vi "update anott. name.vi"(8 "error in (no error)":errorcluster, 9 "Annotation No":i32, 10 "Name":string, 11 "XYGraph in":refnum<vi>) -> (0 "error out":errorcluster, 3 "XYGraph out":refnum<vi>)   [LabVIEW 2014]
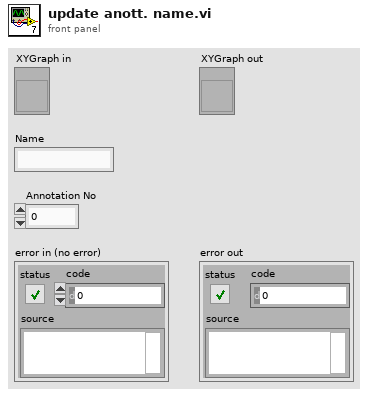
[diagram p1: front panel]
types:
  T1 = typedef "LVAnnotationListTypeDef.ctl" = cluster{"Name":string, "Color":u32, "Style":u8, "Point Style":u8, "Name Visible":bool, "Allow Drag":bool, "Annotation Mode":u32, "Plot":i32, "Index":i32, "Position":cluster{"X":dbl, "Y":dbl}, "X Scale":u32, "Y Scale":u32, "Show Arrow":bool, "Lock Name":bool, "Plot Area":i32, "Label Offset":cluster{"X":dbl, "Y":dbl}}[]
  T2 = cluster{"Name":string, "Color":u32, "Style":u8, "Point Style":u8, "Name Visible":bool, "Allow Drag":bool, "Annotation Mode":u32, "Plot":i32, "Index":i32, "Position":cluster{"X":dbl, "Y":dbl}, "X Scale":u32, "Y Scale":u32, "Show Arrow":bool, "Lock Name":bool, "Plot Area":i32, "Label Offset":cluster{"X":dbl, "Y":dbl}}
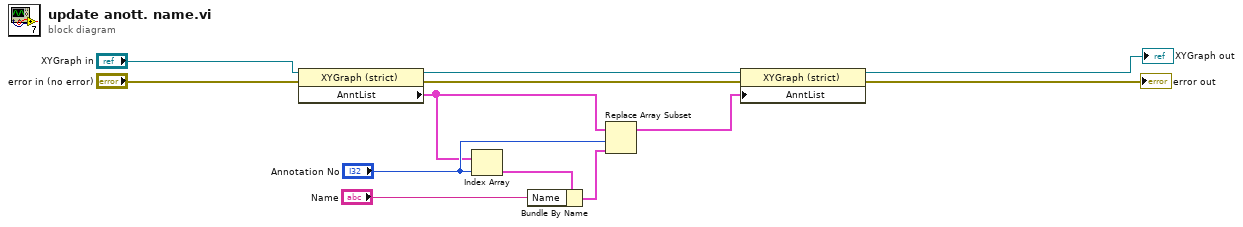
[diagram p0: block diagram]
diagram:
  n1 = property class="XYGraph (strict)"(reference="XYGraph in", error in="error in (no error)") -> (reference out=w8:refnum<vi>, error out=w7:errorcluster, "AnntList"=w4:T1)
  n2 = Index Array(array=w4, index="Annotation No") -> (element=w9:T2)
  n3 = Bundle By Name(cluster=w9, "Name"="Name") -> (w10:T2)
  n4 = Replace Array Subset "Replace Array Subset"(array=w4, new element=w10, index="Annotation No") -> (w5:T1)
  n5 = property class="XYGraph (strict)"(reference=w8, error in=w7, "AnntList"=w5) -> (reference out=→"XYGraph out":refnum<vi>, error out=→"error out":errorcluster)
